vi "process_data.vi"(0 "abstract_dataprocessing_base in":refnum<class "abstract_dataprocessing_base.lvclass">, 5 "datas":refnum<class "abstract_data_base.lvclass">[](array[class]), 11 "error in (no error)":errorcluster) -> (4 "abstract_dataprocessing_base out":refnum<class "abstract_dataprocessing_base.lvclass">, 6 "nodes":refnum<class "data_node.lvclass">[](array[class]), 15 "error out":errorcluster)   [LabVIEW 2020, in "abstract_dataprocessing_base.lvclass"]
uses:
  abstract_dataprocessing_base.lvclass
  data/abstract_data_base/abstract_data_base.lvclass
  data/data_node/data_node.lvclass
  D:/Personal/LabVIEW LLMs/src/data/abstract_data_base/abstract_data_base.lvclass
  data/data_document/data_document.lvclass
  3406f82f-4656-4d5d-a0f8-6c99c24468b1.vi
  <vilib>/Comparison/Equal/Equal Functor/Equal Functor.lvclass
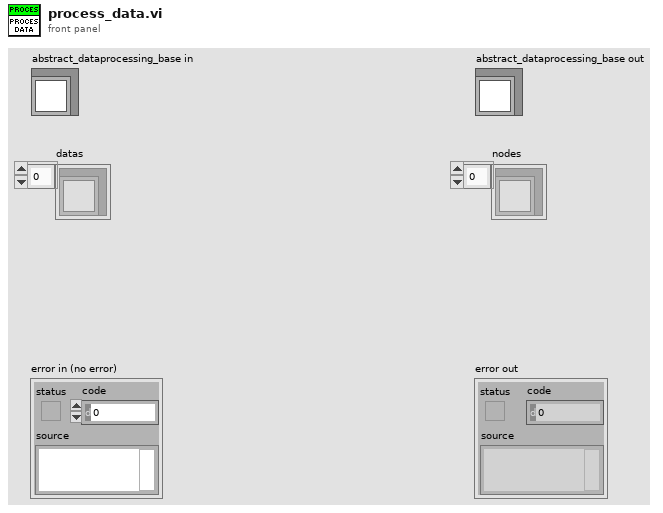
[diagram p1: front panel]
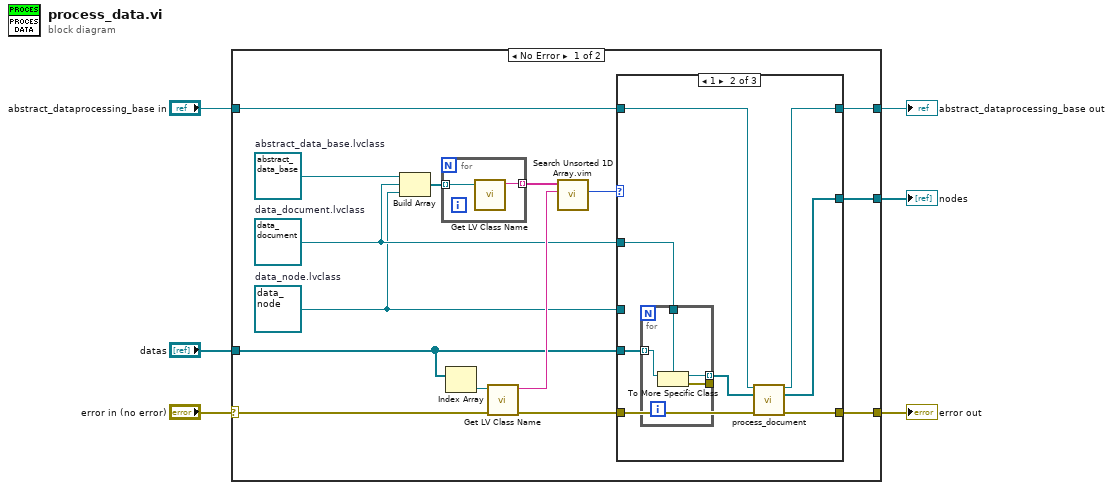
[diagram p0: block diagram]
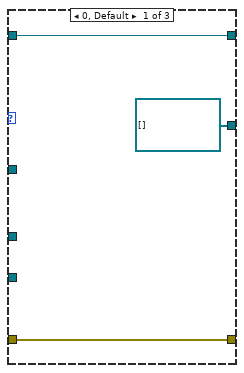
[diagram p2: hidden frame]
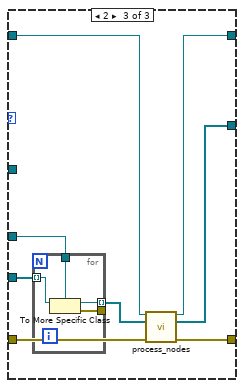
[diagram p3: hidden frame]
diagram:
  n1 = case shown="No Error" "error in (no error)" {
    selector: "error in (no error)" -> [w21 w52]
    tunnel: [w13 w52] -> w5
    tunnel: [w11 w51] -> w3
    tunnel: "abstract_dataprocessing_base in" -> [w12 w51]
    tunnel: "datas" -> [w10 _]
    tunnel: [w8 _] -> w1
    frame No Error {
      w7 = refnum<class "data_node.lvclass"> refnum  # data_node.lvclass
      w9 = refnum<class "data_document.lvclass"> refnum  # data_document.lvclass
      w19 = refnum<class "abstract_data_base.lvclass"> refnum  # abstract_data_base.lvclass
      n2 = Build Array(w19, w9, w7) -> (w18:refnum<class "abstract_data_base.lvclass">[])
      n3 = for {
        tunnel: w18 -> [w50] mode=indexing
        tunnel: [w49] -> w17 mode=indexing
        n4 = call <vilib>:"Get LV Class Name.vi"("object"=w50) -> ("class name"=w49:string)  [unwired: 9 in, 1 out]
      }
      n5 = Index Array(array=w10) -> (element=w20:refnum<class "abstract_data_base.lvclass">)  [unwired: 1 in]
      n6 = call <vilib>:"Get LV Class Name.vi"("error in (no error)"=w21, "object"=w20) -> ("error out"=w15:errorcluster, "class name"=w16:string)  [unwired: 8 in]
      n7 = call "Search Unsorted 1D Array.vim"("element"=w16, "unsorted 1D array"=w17) -> ("index of element"=w14:i32)  [unwired: 9 in]
      n8 = case shown="1" w14 {
        tunnel: w15 -> [w24 w32 w44]
        tunnel: [w24 w31 w43] -> w13
        tunnel: w12 -> [w23 w30 w42]
        tunnel: [w23 w29 w41] -> w11
        tunnel: w10 -> [_ w28 w40]
        tunnel: w9 -> [_ w27 _]
        tunnel: [refnum<class "data_node.lvclass">[] [] ("nodes") w25 w38] -> w8
        tunnel: w7 -> [_ _ w37]
        frame 0, Default {
        }
        frame 1 {
          n9 = for {
            tunnel: w28 -> [w36] mode=indexing
            tunnel: w27 -> [w35]
            tunnel: [w34] -> w26 mode=indexing
            tunnel: [w33] -> _
            n10 = To More Specific Class(target class=w35, reference=w36) -> (specific class reference=w34:refnum<class "data_document.lvclass">, error out=w33:errorcluster)  [unwired: 1 in]
          }
          n11 = call-dynamic "process_document.vi"("abstract_dataprocessing_base in"=w30, "documents"=w26, "error in (no error)"=w32) -> ("abstract_dataprocessing_base out"=w29:refnum<class "abstract_dataprocessing_base.lvclass">, "nodes"=w25:refnum<class "data_node.lvclass">[], "error out"=w31:errorcluster)  [unwired: 10 in]
        }
        frame 2 {
          n12 = for {
            tunnel: w40 -> [w48] mode=indexing
            tunnel: w37 -> [w47]
            tunnel: [w46] -> w39 mode=indexing
            tunnel: [w45] -> _
            n13 = To More Specific Class(target class=w47, reference=w48) -> (specific class reference=w46:refnum<class "data_node.lvclass">, error out=w45:errorcluster)  [unwired: 1 in]
          }
          n14 = call-dynamic "process_nodes.vi"("abstract_dataprocessing_base in"=w42, "nodes"=w39, "error in (no error)"=w44) -> ("abstract_dataprocessing_base out"=w41:refnum<class "abstract_dataprocessing_base.lvclass">, "nodes"=w38:refnum<class "data_node.lvclass">[], "error out"=w43:errorcluster)  [unwired: 10 in]
        }
      }
    }
    frame Error {
    }
  }
  "error out" <- w5
  "abstract_dataprocessing_base out" <- w3
  "nodes" <- w1
